vi "CreerDossiers.vi"(3 "Entrée d'erreur":errorcluster, 5 "NomProjet":string) -> (0 "error out":errorcluster, 2 "NomProjetOut":string)   [LabVIEW 2017]
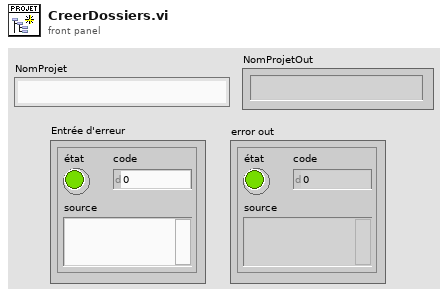
[diagram p1: front panel]
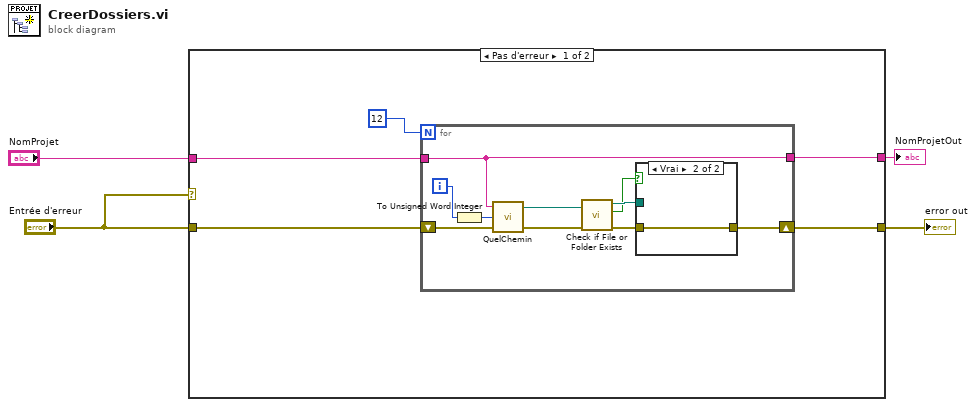
[diagram p0: block diagram]
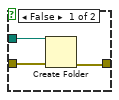
[diagram p2: hidden frame]
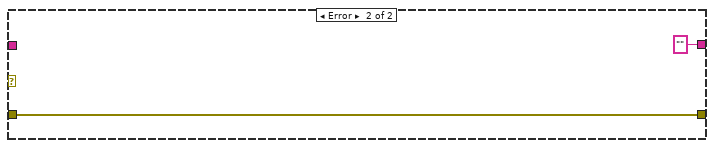
[diagram p3: hidden frame]
diagram:
  n1 = case shown="Pas d'erreur" "Entrée d'erreur" {
    tunnel: "Entrée d'erreur" -> [w7 w25]
    tunnel: [w8 w25] -> w4
    tunnel: "NomProjet" -> [w6 _]
    tunnel: [w5 "" ("NomProjet")] -> w1
    frame No Error {
      n2 = for {
        N: 12 -> [_]
        shift-right: [w13] -> w8
        shift-left: w7 -> [w16]
        tunnel: w6 -> [w12]
        tunnel: [w12] -> w5
        i -> [w11]
        n3 = To Unsigned Word Integer(number=w11) -> (unsigned 16bit integer=w10:u16)
        n4 = call "QuelChemin.vi"("Entrée d'erreur"=w16, "WhichPath?"=w10, "NomProjet"=w12) -> ("Sortie d'erreur"=w15:errorcluster, "SurDisqueLocal"=w14:path)  [unwired: 1 out]
        n5 = call <vilib>:"Check if File or Folder Exists.vi"("error in (no error)"=w15, "path"=w14) -> ("error out"=w18:errorcluster, "file or folder exists?"=w17:bool, "dup path"=w19:path)  [unwired: 7 in]
        n6 = case shown="Vrai" w17 {
          tunnel: w18 -> [w21 w23]
          tunnel: [w20 w23] -> w13
          tunnel: w19 -> [w22 _]
          frame False {
            n7 = Create Folder(path (use dialog)=w22, error in=w21) -> (error out=w20:errorcluster)  [unwired: 1 in, 2 out]
          }
          frame True {
          }
        }
      }
    }
    frame Error {
    }
  }
  "error out" <- w4
  "NomProjetOut" <- w1
